vi "DriveControlerBuffer.vi"(10 "Fast Drive":bool, 11 "Input":dbl) -> (1 "Serializer Out":dbl, 3 "Drive Output":dbl)   [LabVIEW 2016]
uses:
  Robot Global Data.vi
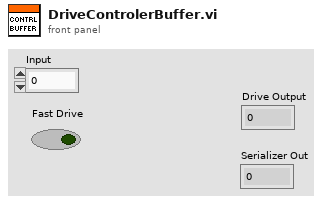
[diagram p1: front panel]
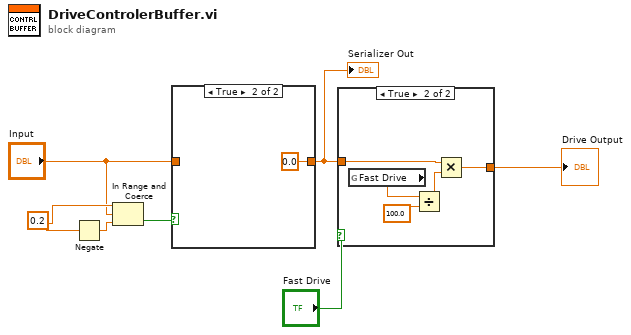
[diagram p0: block diagram]
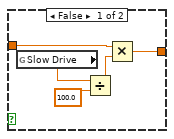
[diagram p2: hidden frame]
diagram:
  w4 = 0.2
  n1 = Negate(x=w4) -> (-x=w5:dbl)
  n2 = In Range and Coerce(upper limit=w4, x="Input", lower limit=w5) -> (In Range?=w7:bool)  [unwired: 1 out]
  n3 = case shown="True" w7 {
    tunnel: [w8 0.0 ("Input")] -> w1
    tunnel: "Input" -> [w8 _]
    frame False {
    }
    frame True {
    }
  }
  "Serializer Out" <- w1
  n4 = case shown="True" "Fast Drive" {
    tunnel: w1 -> [w12 w17]
    tunnel: [w11 w16] -> w2
    frame False {
      n5 = global read "Robot Global Data.vi" "Slow Drive"() -> (w10:dbl)
      n6 = Divide(x=w10, y=100.0) -> (x/y=w14:dbl)
      n7 = Multiply(x=w12, y=w14) -> (x*y=w11:dbl)
    }
    frame True {
      n8 = global read "Robot Global Data.vi" "Fast Drive"() -> (w15:dbl)
      n9 = Divide(x=w15, y=100.0) -> (x/y=w19:dbl)
      n10 = Multiply(x=w17, y=w19) -> (x*y=w16:dbl)
    }
  }
  "Drive Output" <- w2
